vi "open samples data 2.vi"() -> (3 "Sample cluster":T1={"General description"="", "Sample setup"={"integration time"=0.5, "rinse time"=10.0, "sample time"=10.0, "sample type"=0}, "Absorbance"=[], "Analyst"="", "Sample descriptions"=[], "good data"=[]} {"Absorbance" format="%.2e"; "Sample setup"."sample type" items=["Sample Cuvet", "Sipper Cell", "No Dialog"]; "Sample setup"."sample time" min=0.0 max=100.0 step=1.0 format="%.1f"; "Sample setup"."rinse time" min=0.0 max=100.0 step=1.0 format="%.1f"; "Sample setup"."integration time" format="%.1f"})   [LabVIEW 2015]
uses:
  sample cluster.ctl
  settings.ctl
  file/file action.ctl
panel:
  out "canceled":bool
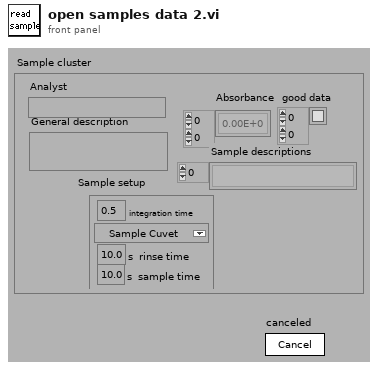
[diagram p1: front panel]
types:
  T1 = typedef "sample cluster.ctl" = cluster{"General description":string, "Sample setup":T2, "Absorbance":dbl[][], "Analyst":string, "Sample descriptions":string[], "good data":bool[][]}
  T2 = typedef "settings.ctl" = cluster{"integration time":sgl, "rinse time":dbl[unit], "sample time":dbl[unit], "sample type":u16}
  T3 = typedef "file action.ctl" = enum16{"Save", "Open"}
  T4 = enum16{"open", "open or create", "create or replace", "create", "open (read only)"}
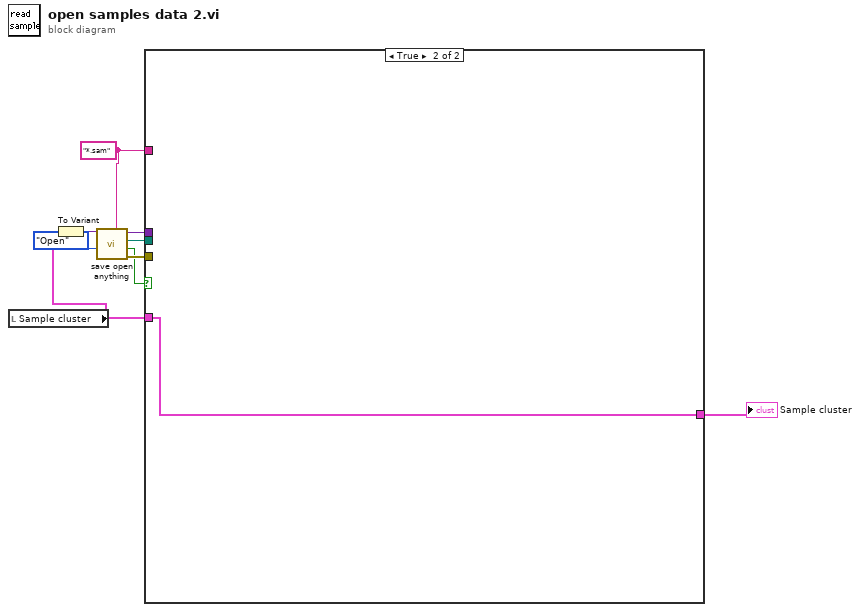
[diagram p0: block diagram]
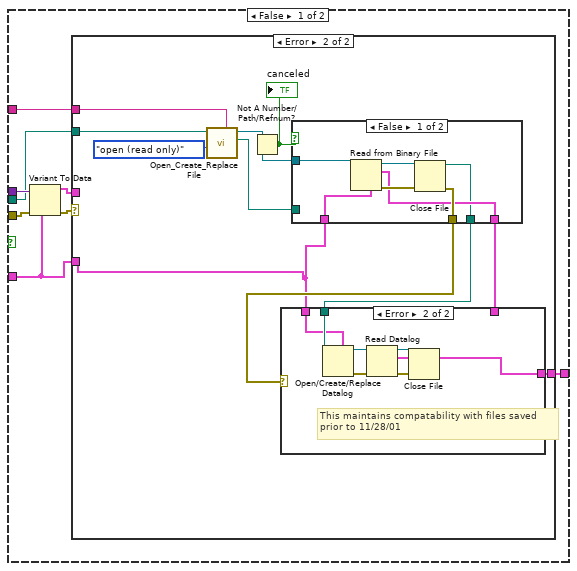
[diagram p2: hidden frame]
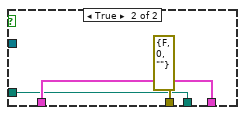
[diagram p5: hidden frame]
diagram:
  w2 = "*.sam" ("pattern")
  n1 = local read "Sample cluster"() -> (w3:T1)
  n2 = To Variant(anything=w3) -> (Variant=w8:variant)
  n3 = call "save open anything.vi"("Variant"=w8, "Action"=file_action."Open", "pattern"=w2) -> ("Variant out"=w6:variant, "new file path"=w4:path, "canceled"=w1:bool, "error out"=w7:errorcluster)  [unwired: 4 in]
  n4 = case shown="True" w1 {
    tunnel: [w17 w48] -> w9
    tunnel: w7 -> [w16 _]
    tunnel: w6 -> [w15 _]
    tunnel: w4 -> [w13 _]
    tunnel: w3 -> [w11 w48]
    tunnel: w2 -> [w10 _]
    frame False {
      n5 = Variant To Data(error in=w16, type=w11, Variant=w15) -> (data=w12:T1, error out=w14:errorcluster)
      n6 = case shown="Error" w14 {
        tunnel: [w18 w23] -> w17
        tunnel: w11 -> [_ w21]
        tunnel: w10 -> [_ w20]
        tunnel: w13 -> [_ w19]
        tunnel: w12 -> [w18 _]
        frame No Error {
        }
        frame Error {
          n7 = call <vilib>:"Open_Create_Replace File.vi"("pattern"=w20, "function (open:0)"=T4."open (read only)", "file path"=w19) -> ("new file path"=w24:path, "refnum"=w28:refnum<file>)  [unwired: 5 in, 2 out]
          n8 = Not A Number/Path/Refnum?(number/path/refnum=w28) -> (NaN/Path/Refnum?=w22:bool)
          "canceled" <- w22
          n9 = case shown="False" w22 {
            tunnel: w28 -> [w42 _]
            tunnel: w21 -> [w41 w46]
            tunnel: [w40 errorcluster {"status"=FALSE, "code"=0, "source"=""} ("error out")] -> w27
            tunnel: [w39 w46] -> w26
            tunnel: [w38 w45] -> w25
            tunnel: w24 -> [_ w45]
            frame False {
              n10 = Read from Binary File(5:w41, 11:w42) -> (0:w43:errorcluster, 2:w39:T1, 3:w44:refnum<file>)  [unwired: 4 in, 1 out]
              n11 = Close File(refnum=w44, error in=w43) -> (path=w38:path, error out=w40:errorcluster)
            }
            frame True {
            }
          }
          n12 = case shown="Error" w27 {
            tunnel: [w30 w37] -> w23
            tunnel: w26 -> [w30 _]
            tunnel: w25 -> [_ w32]
            tunnel: w21 -> [_ w31]
            frame No Error {
            }
            frame Error {
              # "This maintains compatability with files saved \nprior to 11/28/01"
              n13 = Open/Create/Replace Datalog(5:w31, 11:w32) -> (0:w34:errorcluster, 3:w35:refnum<k1>)  [unwired: 4 in, 1 out]
              n14 = Read Datalog(4:w34, 7:w35) -> (0:w33:errorcluster, 2:w37:T1, 3:w36:refnum<k1>)  [unwired: 1 in]
              n15 = Close File(refnum=w36, error in=w33) -> ()  [unwired: 2 out]
            }
          }
        }
      }
    }
    frame True {
    }
  }
  "Sample cluster" <- w9
